vi "Conclude Call.vi"(8 "error in":errorcluster, 11 "ASE Handle":refnum<class "ase.lvclass">) -> (0 "error out":errorcluster, 1 "Exit Code":i32, 3 "Event References":T1)   [LabVIEW 2020, in "ase.lvlib" / "ase.lvclass"]
doc: "<B>Conclude the Asynchronous System Exec call.</B>\n\nThis VI waits for the call to finish and then deallocates internal resources.\n\n<B>This VI will still operate when there is an error at the error-in terminal.</B>\n\nThis VI generates the following errors:\n-5691000: Internal Library Error. Check Error Message for more details.\n1556: Invalid Handle Supplied"
uses:
  ase.lvclass
  ase.lvclass/ase.ctl
  bin/ase_32-3.dll
  Standard Error.ctl
  Standard Output.ctl
  Did Exit.ctl
  Event References.ctl
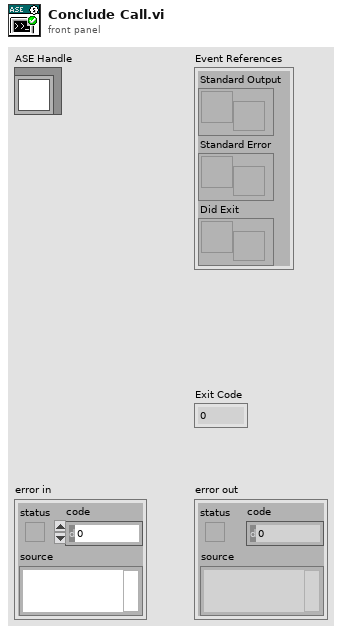
[diagram p1: front panel]
types:
  T1 = typedef "ase.lvlib/ase.lvclass/Event References.ctl" = cluster{"Standard Output":refnum<user-event>, "Standard Error":refnum<user-event>, "Did Exit":refnum<user-event>}
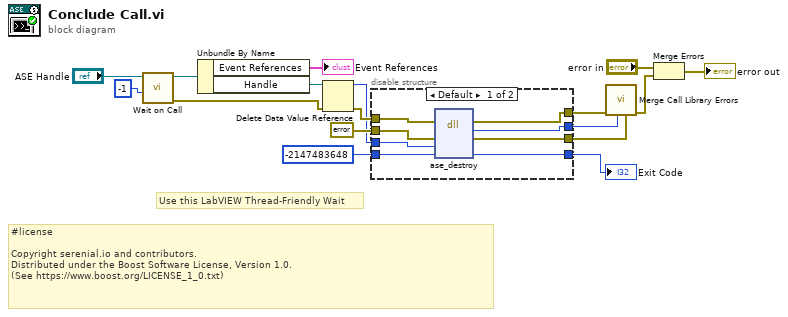
[diagram p0: block diagram]
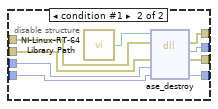
[diagram p2: hidden frame]
diagram:
  # "Use this LabVIEW Thread-Friendly Wait"
  # "#license\n\nCopyright serenial.io and contributors.\nDistributed under the Boost Software License, Version 1.0.\n(See https://www.boost.org/LICENSE_1_0.txt)"
  n1 = call "Wait on Call.vi"("Timeout (ms)"=-1, "ASE Handle"="ASE Handle") -> ("error out"=w2:errorcluster, "ASE Handle Duplicate"=w3:refnum<class "ase.lvclass">)  [unwired: 7 in, 1 out]
  n2 = Unbundle By Name(w3) -> ("Event References"=→"Event References":T1, "Handle"=w12:refnum<data-value>)
  n3 = Delete Data Value Reference(data value reference=w12, error in=w2) -> (data value=w9:u64, error out=w11:errorcluster)
  n4 = disable-structure "Conditional Disable Structure" shown="Default" {
    disable-tunnel: w11 -> [w25 w34]
    disable-tunnel: errorcluster {"status"=FALSE, "code"=0, "source"=""} ("error") -> [w24 w32]
    disable-tunnel: w9 -> [w18 w31]
    disable-tunnel: [w20 w33] -> w8
    disable-tunnel: [w19 w27] -> w7
    disable-tunnel: [w21 w28] -> w6
    disable-tunnel: [w22 w29] -> w5
    disable-tunnel: -2147483648 ("exit_code") -> [w23 w30]
    frame condition #0 (active) {
      n5 = dll-call lib="C:/serenial/lib/asynchronous-system-exec/LabVIEW/ase/ase/bin/ase_*-3.*" fn="ase_destroy" ("AsyncSystemExec*.*:wrapperVersion")(error in=w25, "Error Out"=w24, "process"=w18, "exit_code"=w23) -> (error out=w20:errorcluster, "Error Code"=w19:i32, "Error Out"=w21:errorcluster, "exit_code"=w22:i32)  [unwired: 3 in, 1 out]
    }
    frame condition #1 {
      n6 = call "NI-Linux-RT-64 Library Path.vi"() -> ("Path"=w26:path)
      n7 = dll-call lib="?" fn="ase_destroy" ("AsyncSystemExec*.*:wrapperVersion")(path in=w26, error in=w34, "Error Out"=w32, "process"=w31, "exit_code"=w30) -> (error out=w33:errorcluster, "Error Code"=w27:i32, "Error Out"=w28:errorcluster, "exit_code"=w29:i32)  [unwired: 2 in, 1 out]
    }
  }
  "Exit Code" <- w5
  n8 = call "Merge Call Library Errors.vi"("Library Call Returned Error"=w6, "Error Code"=w7, "error in"=w8) -> ("error IO"=w15:errorcluster)  [unwired: 8 in]
  n9 = Merge Errors("error in", w15) -> (→"error out":errorcluster)
